vi "uObserver_Registration.vi"(8 "error in (no error)":errorcluster, 11 "uObserver in":refnum<class "uObserver.lvclass">) -> (0 "error out":errorcluster, 3 "uObserver out":refnum<class "uObserver.lvclass">)   [LabVIEW 2021, in "uFramework_pack_uActor.lvlib" / "uObserver.lvclass"]
doc: "Dynamic dispatch method to allow children Observers to override the initial Pub/Sub registration behavior.\n<B>This is called before the uActor's Init method.</B> If the registration returns an error, the observer actor will fail to launch and will not invoke the uActor ErrHandling method. It will just return a nested-actor-stop message to the caller.\n\n<B>This method registers the observer actor as both a publisher and a subscriber. It uses the registration policies in the object private data.</B> These may be passed in by the caller during the actor launch or may be determined by the concrete implementation of the observer child. When the latter is the case, the recommended implementation is to create an override for the uObserver_Registration method, then use the accessor methods to update/manipulate the policy then call the parent method downstream."
uses:
  uObserver.lvclass
  uObserver.lvclass/uObserver.ctl
  Bin/uFramework.lvlibp/uTransport_uActor/uTransport_uActor.lvclass
  U:/Projects/uFramework/Bin/uFramework.lvlibp/uTransport/uTransport.lvclass
  Bin/uStringManipulation.lvlibp/uFramework/uStringManipulation/uStringManipulation.lvclass
  Bin/uFramework.lvlibp/uPolicy/uPolicy.lvclass
  Bin/uFramework.lvlibp/uClient_Publisher/uClient_Publisher.lvclass
  Bin/uFramework.lvlibp/uClient_Subscriber/uClient_Subscriber.lvclass
  Bin/uFramework.lvlibp/uActor/uActor.lvclass
  U:/Projects/uFramework/Bin/uFramework.lvlibp/uActor/uActor.lvclass
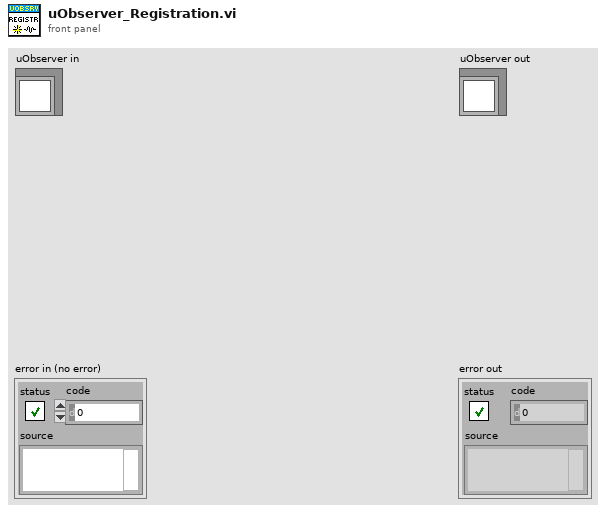
[diagram p1: front panel]
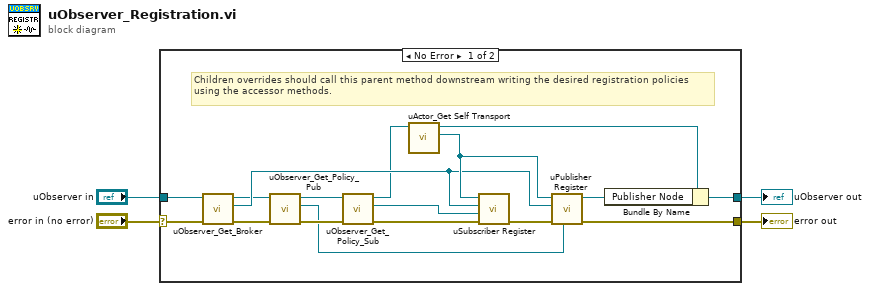
[diagram p0: block diagram]
diagram:
  n1 = case shown="No Error" "error in (no error)" {
    selector: "error in (no error)" -> [w11 w23]
    tunnel: [w14 w23] -> w3
    tunnel: [w5 w22] -> w1
    tunnel: "uObserver in" -> [w8 w22]
    frame No Error {
      # "Children overrides should call this parent method downstream writing the desired registration policies using the accessor methods."
      n2 = call "uObserver_Get_Broker.vi"("error in (no error)"=w11, "uObserver in"=w8) -> ("error out"=w21:errorcluster, "Broker's Transport"=w16:refnum<class "uTransport_uActor.lvclass">, "uObserver out"=w12:refnum<class "uObserver.lvclass">)  [unwired: 7 in]
      n3 = call "uObserver_Get_Policy_Pub.vi"("error in (no error)"=w21, "uObserver in"=w12) -> ("error out"=w20:errorcluster, "uStringManipulation"=w17:refnum<class "uStringManipulation.lvclass">, "uObserver out"=w13:refnum<class "uObserver.lvclass">)  [unwired: 7 in]
      n4 = call "uObserver_Get_Policy_Sub.vi"("error in (no error)"=w20, "uObserver in"=w13) -> ("error out"=w10:errorcluster, "uPolicy"=w18:refnum<class "uPolicy.lvclass">, "uObserver out"=w9:refnum<class "uObserver.lvclass">)  [unwired: 7 in]
      n5 = call "uActor_Get Self Transport.vi"("uActor in"=w9) -> ("Actor Transport"=w19:refnum<class "uTransport_uActor.lvclass">, "uActor out"=w6:refnum<class "uObserver.lvclass">)  [unwired: 9 in]
      n6 = call "uSubscriber Register.vi"("error in (no error)"=w10, "Policy (All-Topics)"=w18, "Broker"=w16, "Subscriber's uTransport"=w19) -> ("error out"=w15:errorcluster)  [unwired: 7 in]
      n7 = call "uPublisher Register.vi"("uStringManipulation"=w17, "error in (no error)"=w15, "Broker"=w16, "Publisher's uTransport"=w19) -> ("error out"=w14:errorcluster, "uClient_Publisher out"=w7:refnum<class "uClient_Publisher.lvclass">)  [unwired: 6 in]
      n8 = Bundle By Name(cluster=w6, "Publisher Node"=w7) -> (w5:refnum<class "uObserver.lvclass">)
    }
    frame Error {
    }
  }
  "error out" <- w3
  "uObserver out" <- w1
